vi "dispose client.vi"(8 "error in":errorcluster, 11 "lvlibretls client socket in":refnum<class "lvlibretls client socket.lvclass">) -> (0 "error out":errorcluster)   [LabVIEW 2016, in "lvlibretls client socket.lvclass"]
uses:
  lvlibretls client socket.lvclass
  C:/Users/IEUser/Desktop/tlssimple/libretls/context parent/lvlibretls configurable context.lvclass
  context parent/lvlibretls configurable context.lvclass
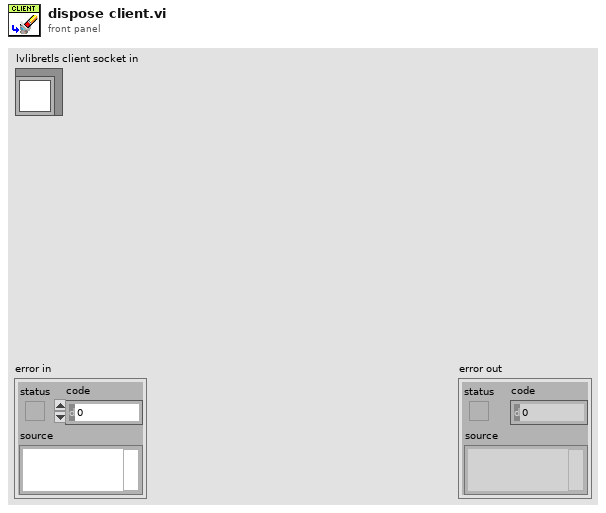
[diagram p1: front panel]
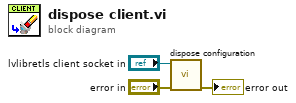
[diagram p0: block diagram]
diagram:
  n1 = call "dispose configuration.vi"("error in"="error in", "lvlibretls configurable context in"="lvlibretls client socket in") -> ("error out"=→"error out":errorcluster)  [unwired: 9 in]
